vi "GetCameraInfo.vi"(7 "LabVIEW Web Service Request":refnum<class "Web Request.lvclass">) -> ()   [LabVIEW 2017]
uses:
  <vilib>/wsapi/Web Request.lvclass
  DataAccessors/action.ctl
  DataAccessors/VisionWebServiceData.lvlib
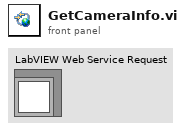
[diagram p1: front panel]
types:
  T1 = typedef "VisionWebServiceData.lvlib/action.ctl" = enum16{"Get", "Set"}
  T2 = typedef "IrManageCameras.lvlib/camera.ctl" = cluster{"InterfaceName":string, "VendorName":string, "ModelName":string, "CameraFileName":string, "SerialNumber":string, "IP Address":string, "PhysicalPort":string, "CameraName":string, "ChannelId":string, "CameraId":string, "InDeviceModel":bool}
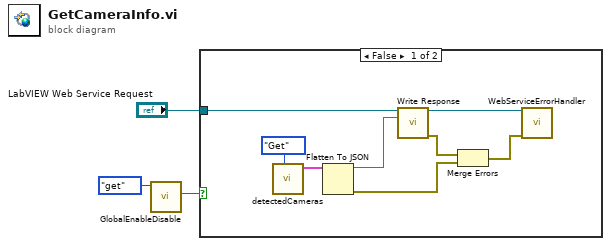
[diagram p0: block diagram]
diagram:
  n1 = call "GlobalEnableDisable.vi"("action"=enum16{"init", "set", "get"}."get") -> ("DisableDeviceWebService"=w1:bool)  [unwired: 10 in]
  n2 = case shown="False" w1 {
    tunnel: "LabVIEW Web Service Request" -> [w10 _]
    frame False {
      n3 = call "detectedCameras.vi"("action"=action."Get") -> ("Discovered Cameras"=w9:T2[])  [unwired: 9 in, 1 out]
      n4 = Flatten To JSON(anything=w9) -> (JSON string=w7:string, 11:w5:errorcluster)  [unwired: 2 in]
      n5 = call <vilib>:"Write Response.vi"("LabVIEW Web Service Request"=w10, "response string"=w7) -> ("LabVIEW Web Service Request out"=w11:refnum<class "Web Request.lvclass">, "error out"=w6:errorcluster)  [unwired: 12 in]
      n6 = Merge Errors(w6, w5) -> (w4:errorcluster)
      n7 = call "WebServiceErrorHandler.vi"("LabVIEW Web Service Request"=w11, "error in (no error)"=w4) -> ()  [unwired: 12 in, 2 out]
    }
    frame True {
    }
  }
